vi "test-trajectory-transform-same-shape-verify.vi"(9 "TrajStates2":T1[](array[typedef]) {"POSE"."ROTATION"."SIN" format="%13.4f"; "POSE"."ROTATION"."COS" format="%13.4f"; "POSE"."ROTATION"."VALUE" format="%13.4f"; "POSE"."TRANSLATION"."Y" format="%14.3f"; "POSE"."TRANSLATION"."X" format="%14.3f"}, 11 "TrajStates1":T1[](array[typedef]) {"POSE"."ROTATION"."SIN" format="%13.4f"; "POSE"."ROTATION"."COS" format="%13.4f"; "POSE"."ROTATION"."VALUE" format="%13.4f"; "POSE"."TRANSLATION"."Y" format="%14.3f"; "POSE"."TRANSLATION"."X" format="%14.3f"}) -> (3 "SameShape":bool)   [LabVIEW 2019]
uses:
  <vilib>/Rock Robotics/WPI/ThirdParty/JAS_Junk/TrajLib/TRAJ_STATE.ctl
  <vilib>/Rock Robotics/WPI/ThirdParty/JAS_Junk/TrajLib/POSE2D.ctl
  <vilib>/Rock Robotics/WPI/ThirdParty/JAS_Junk/TrajLib/TRANSLATION2D.ctl
  <vilib>/Rock Robotics/WPI/ThirdParty/JAS_Junk/TrajLib/ROTATION2D.ctl
  <vilib>/Rock Robotics/WPI/ThirdParty/JAS_Junk/TrajLib/Transform_Create_PosePose.vi
  <vilib>/Rock Robotics/WPI/ThirdParty/JAS_Junk/TrajLib/Pose_New_TRRO.vi
  <vilib>/Rock Robotics/WPI/ThirdParty/JAS_Junk/TrajLib/Translation_Equals.vi
  <vilib>/Rock Robotics/WPI/ThirdParty/JAS_Junk/TrajLib/Rotation_Equals.vi
  <vilib>/Rock Robotics/WPI/ThirdParty/JAS_Junk/TrajLib/Rotation_UnaryMinus.vi
  <vilib>/Rock Robotics/WPI/ThirdParty/JAS_Junk/TrajLib/Translation_RotateBy.vi
  <vilib>/Rock Robotics/WPI/ThirdParty/JAS_Junk/TrajLib/Translation_Minus.vi
  <vilib>/Rock Robotics/WPI/ThirdParty/JAS_Junk/TrajLib/Rotation_Minus.vi
  <vilib>/Rock Robotics/WPI/ThirdParty/JAS_Junk/TrajLib/Util_CalcDist.vi
  <vilib>/Rock Robotics/WPI/ThirdParty/JAS_Junk/TrajLib/Rotation_CreateAngle.vi
  <vilib>/Rock Robotics/WPI/ThirdParty/JAS_Junk/TrajLib/Translation_Create.vi
  <vilib>/Rock Robotics/WPI/ThirdParty/JAS_Junk/TrajLib/Rotation_RotateBy.vi
  <vilib>/Rock Robotics/WPI/ThirdParty/JAS_Junk/TrajLib/Rotation_CreateXY.vi
  <vilib>/Rock Robotics/WPI/ThirdParty/JAS_Junk/TrajLib/Trajectory_Library.lvlib
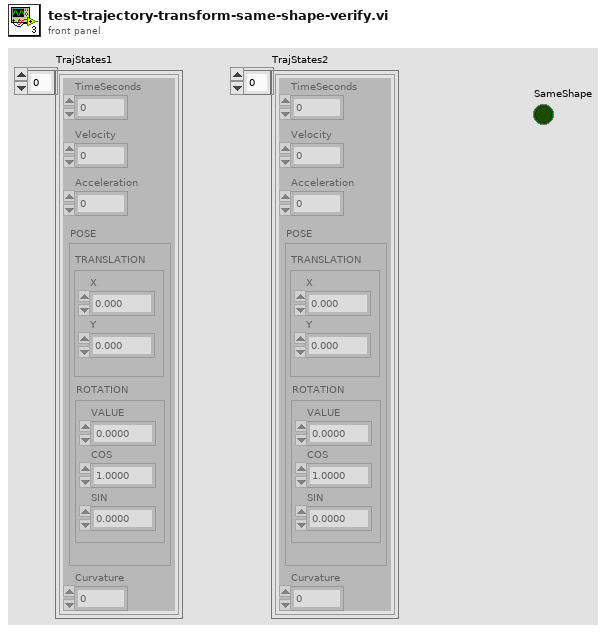
[diagram p1: front panel]
types:
  T1 = typedef "Trajectory_Library.lvlib/TRAJ_STATE.ctl" = cluster{"TimeSeconds":dbl, "Velocity":dbl, "Acceleration":dbl, "POSE":T2, "Curvature":dbl}
  T2 = typedef "Trajectory_Library.lvlib/POSE2D.ctl" = cluster{"TRANSLATION":T3, "ROTATION":T4}
  T3 = typedef "Trajectory_Library.lvlib/TRANSLATION2D.ctl" = cluster{"X":dbl, "Y":dbl}
  T4 = typedef "Trajectory_Library.lvlib/ROTATION2D.ctl" = cluster{"VALUE":dbl, "COS":dbl, "SIN":dbl}
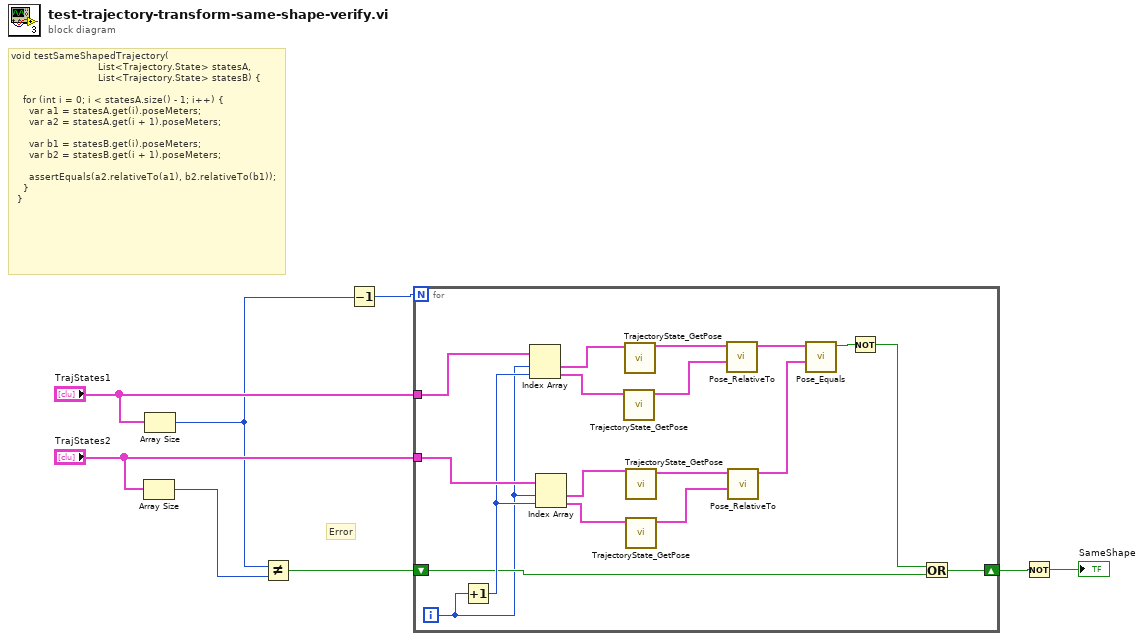
[diagram p0: block diagram]
diagram:
  # "Error"
  # "void testSameShapedTrajectory(\n                             List<Trajectory.State> statesA, \n                             List<Trajectory.State> statesB) {\n\n    for (int i = 0; i < statesA.size() - 1; i++) {\n      var a1 = statesA.get(i).poseMeters;\n      var a2 = statesA.get(i + 1).poseMeters;\n\n      var b1 = statesB.get(i).poseMeters;\n      var b2 = statesB.get(i + 1).poseMeters;\n\n      assertEquals(a2.relativeTo(a1), b2.relativeTo(b1));\n    }\n  }"
  n1 = Array Size(array="TrajStates2") -> (size(s)=w4:i32)
  n2 = Array Size(array="TrajStates1") -> (size(s)=w2:i32)
  n3 = Not Equal?(x=w2, y=w4) -> (x != y?=w3:bool)
  n4 = Decrement(x=w2) -> (x-1=w1:i32)
  n5 = for {
    N: w1 -> [_]
    tunnel: "TrajStates1" -> [w26]
    tunnel: "TrajStates2" -> [w25]
    shift-right: [w15] -> w7
    shift-left: w3 -> [w14]
    i -> [w13]
    n6 = Increment(x=w13) -> (x+1=w24:i32)
    n7 = Index Array(array=w26, index #1=w13, index #2=w24) -> (element #1=w23:T1, element #2=w22:T1)
    n8 = Index Array(array=w25, index #1=w13, index #2=w24) -> (element #1=w21:T1, element #2=w20:T1)
    n9 = call <vilib>:"TrajectoryState_GetPose.vi"("TRAJ_STATE"=w22) -> ("TrajStatePose"=w11:T2)  [unwired: 10 in]
    n10 = call <vilib>:"TrajectoryState_GetPose.vi"("TRAJ_STATE"=w23) -> ("TrajStatePose"=w12:T2)  [unwired: 10 in]
    n11 = call <vilib>:"TrajectoryState_GetPose.vi"("TRAJ_STATE"=w21) -> ("TrajStatePose"=w10:T2)  [unwired: 10 in]
    n12 = call <vilib>:"TrajectoryState_GetPose.vi"("TRAJ_STATE"=w20) -> ("TrajStatePose"=w9:T2)  [unwired: 10 in]
    n13 = call <vilib>:"Pose_RelativeTo.vi"("other POSE"=w11, "in POSE"=w12) -> ("out POSE"=w19:T2)  [unwired: 9 in]
    n14 = call <vilib>:"Pose_RelativeTo.vi"("other POSE"=w9, "in POSE"=w10) -> ("out POSE"=w18:T2)  [unwired: 9 in]
    n15 = call <vilib>:"Pose_Equals.vi"("other POSE"=w18, "in POSE"=w19) -> ("Equals"=w17:bool)  [unwired: 9 in]
    n16 = Not(x=w17) -> (.not. x?=w16:bool)
    n17 = Or(x=w16, y=w14) -> (x .or. y?=w15:bool)
  }
  n18 = Not(x=w7) -> (.not. x?=→"SameShape":bool)
